vi "Page_Source_WriteShared.vi"(6 "ctlReferences":T1, 7 "top tree items":string[](array[string]), 8 "error in (no error)":errorcluster, 10 "AB_Source in":refnum<class "AB_Source.lvclass">[](array[class]), 11 "AB_PackedLibrary in":refnum<class "AB_PackedLibrary.lvclass">) -> (0 "error out":errorcluster, 2 "AB_Source out":refnum<class "AB_Source.lvclass">[](array[class]), 3 "AB_PackedLibrary out":refnum<class "AB_PackedLibrary.lvclass">)   [LabVIEW 2020, in "AB_PackedLibrary.lvclass"]
uses:
  <vilib>/AppBuilder/AB_Classes/PackedLib/AB_PackedLibrary.lvclass
  e:/builds/penguin/labview/branches/2020/dev/dist/vi.lib/AppBuilder/AB_Classes/Build/AB_Build.lvclass
  e:/builds/penguin/labview/branches/2020/dev/dist/vi.lib/AppBuilder/AB_Classes/TargetFile/AB_Targetfile.lvclass
  <resource>/Framework/Providers/Builds/AppBuilder/AB_UI_Page_Source_Files_References.ctl
  <vilib>/AppBuilder/AB_Classes/Source/AB_Source.lvclass
  <resource>/Framework/Providers/Common/provcom_StringGlobals.vi
  <vilib>/AppBuilder/AB_Classes/Build/AB_Build.lvclass
  <vilib>/AppBuilder/AB_Classes/TargetFile/AB_Targetfile.lvclass
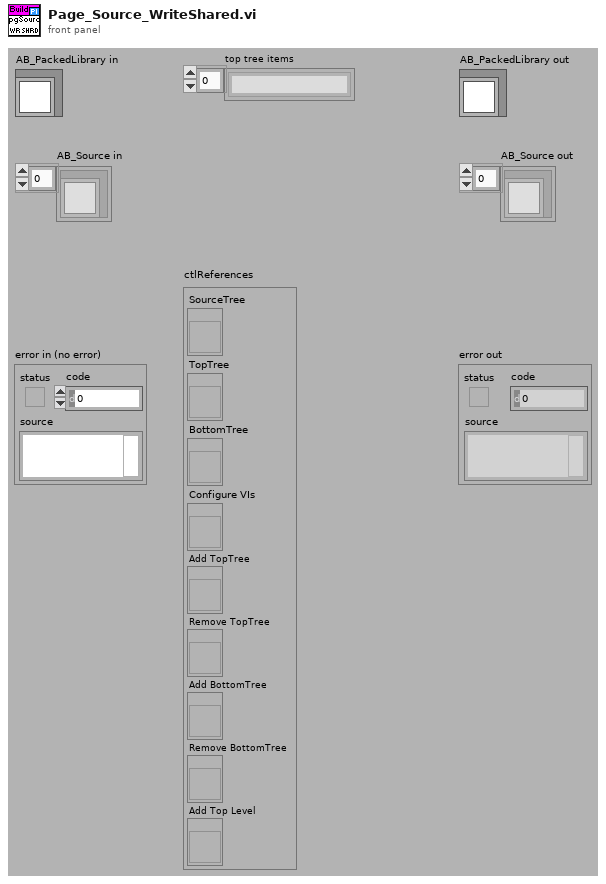
[diagram p1: front panel]
types:
  T1 = typedef "AB_UI_Page_Source_Files_References.ctl" = cluster{"SourceTree":refnum<vi>, "TopTree":refnum<vi>, "BottomTree":refnum<vi>, "Configure VIs":refnum<vi>, "Add TopTree":refnum<vi>, "Remove TopTree":refnum<vi>, "Add BottomTree":refnum<vi>, "Remove BottomTree":refnum<vi>, "Add Top Level":refnum<vi>}
  T2 = typedef "AB_Build.ctl" = cluster{"buildSpecName":string, "buildSpecDescription":string, "destinations":refnum<class "AB_Destination.lvclass">[], "exclusionOption":T3, "defaultLanguage":string, "supportedLanguages":string[], "excludedDirectories":path[], "buildContext":refnum<vi>, "buildObject":T4, "preview":bool, "programatic":bool, "progressBarEvents":T5, "userLog_Path":path, "preActionID":string, "preAction_Path":path, "postActionID":string, "postAction_Path":path, "eng_checkForBrokenVIs?":bool, "eng_verboseLinkerErrors?":bool, "localDest_Path":path, "targetDest_Path":path, "removeVIObject":u16, "cache":refnum<class "PreviewCache.lvclass">, "use cache":bool, "previewCache_ID":string, "buildCache_ID":string, "eng_TempLocalDest_Path":path, "eng_collectDependencies?":bool, "versionInfo":cluster{"buildVersion":cluster{"major":u16, "minor":u16, "patch":u16, "build":u16}, "autoIncrement":bool}, "eng_enableVIChecksums":bool}
  T3 = typedef "AB_Exclusion_Option.ctl" = cluster{"typedefs":bool, "polymorphicVIs":bool, "unusedLibraryItems":bool, "modifyLibraryFile":bool, "edit-timeDependencies":bool, "inlineVIs":bool, "dependent PPLs":bool, "dependent DLLs":bool}
  T4 = typedef "ItemRef.ctl" = u64
  T5 = typedef "provcom_ProgressBar_Events.ctl" = cluster{"newJob":refnum<user-event>, "newItem":refnum<user-event>, "errorMsg":T6, "cancel":refnum<user-event>}
  T6 = typedef "mxLvBuildError.ctl" = refnum<user-event>
  T7 = typedef "AB_Targetfile.ctl" = cluster{"targetfileName":string, "targetfileGUID":string, "enableDebugging":bool, "versionInfo":cluster{"productName":string, "legalCopyright":string, "companyName":string, "internalName":string, "fileDescription":string}, "eng_consolidatedTypeInfo":string, "fastFileFormat":bool, "eng_LEIFBuildData":u32, "versionIndependent":bool}
  T8 = typedef "AB_Source.ctl" = cluster{"path":path, "itemID":string, "parentIndex":i32, "sourceInclusion":T9, "destinationIndex":i32, "properties":T10[], "newName":string, "lvfile":bool, "valid":bool, "eng_inBuild":bool, "eng_isNonVILink":bool, "Amalgamation":bool, "Amalgamation Piece":bool, "eng_delimitedName":string, "preventRename":bool}
  T9 = typedef "AB_Source_Inclusion.ctl" = enum16{"IncludeIfReferenced", "Include", "Exclude", "TopLevel"}
  T10 = typedef "AB_Source_Properties.ctl" = cluster{"sourcePropertyType":T11, "value":variant}
  T11 = typedef "AB_Source_Property_Type.ctl" = enum16{"Remove block diagram", "Remove front panel", "Password", "Window has title bar", "Show menu bar", "Show vertical scroll bar", "Show horizontal scroll bar", "Show toolbar", "Show Abort button", "Show fp when called", "Window behavior", "Allow user to close window", "Window run-time position", "Run when opened", "Allow debugging", "Auto error handling", "Generate guard code", "Use stack variables", "Expression folding", "Integer only", "Inline subVI"}
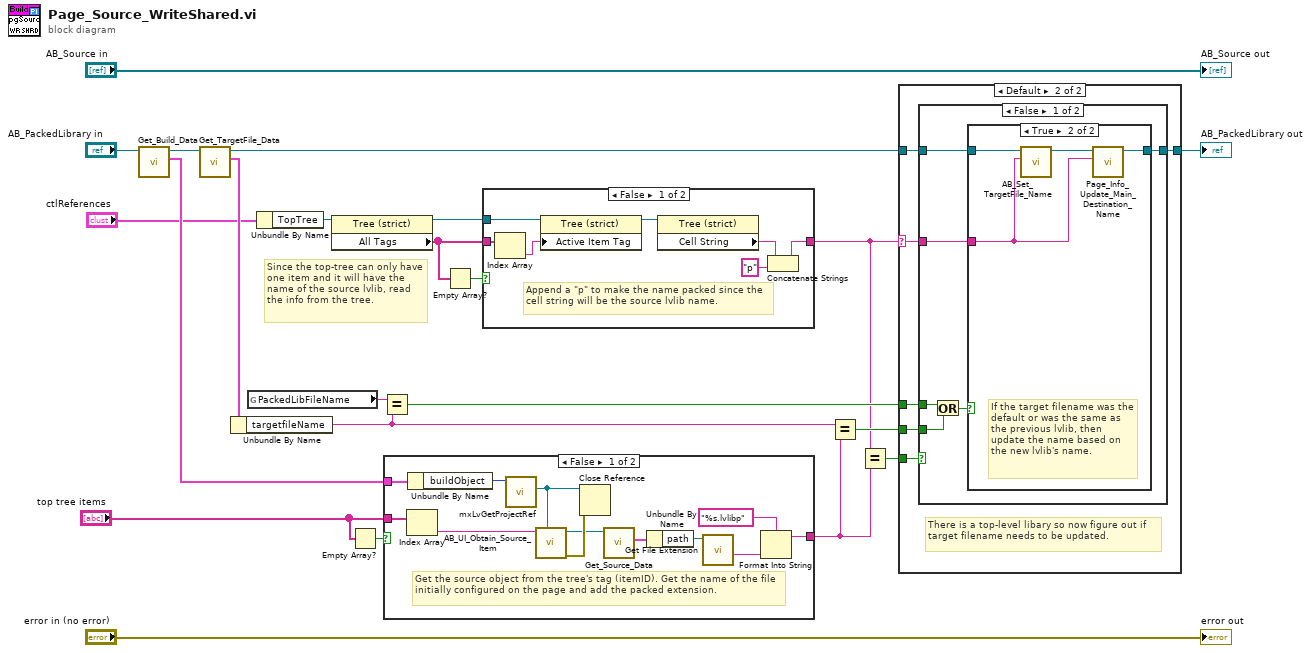
[diagram p0: block diagram]
diagram:
  # "Since the top-tree can only have one item and it will have the name of the source lvlib, read the info from the tree."
  n1 = call <vilib>:"Get_Build_Data.vi"("Class in"="AB_PackedLibrary in") -> ("data"=w18:T2, "Class out"=w17:refnum<class "AB_PackedLibrary.lvclass">)  [unwired: 8 in, 1 out]
  n2 = call <vilib>:"Get_TargetFile_Data.vi"("AB_Targetfile in"=w17) -> ("data"=w16:T7, "AB_Targetfile out"=w7:refnum<class "AB_PackedLibrary.lvclass">)  [unwired: 8 in, 1 out]
  n3 = Unbundle By Name(w16) -> ("targetfileName"=w11:string)
  n4 = global read "provcom_StringGlobals.vi" "PackedLibFileName"() -> (w15:string)
  n5 = Unbundle By Name("ctlReferences") -> ("TopTree"=w4:refnum<vi>)
  n6 = property class="Tree (strict)"(reference=w4) -> (reference out=w3:refnum<vi>, "All Tags"=w2:string[])  [unwired: 1 in, 1 out]
  n7 = Empty Array?(array="top tree items") -> (empty?=w13:bool)
  n8 = Equal?(x=w15, y=w11) -> (x = y?=w12:bool)
  n9 = case shown="False" w13 {
    tunnel: w18 -> [w34 _]
    tunnel: "top tree items" -> [w24 _]
    tunnel: [w23 _] -> w10
    frame False {
      # "Get the source object from the tree's tag (itemID). Get the name of the file initially configured on the page and add the packed extension."
      n10 = Index Array(array=w24) -> (element=w32:string)  [unwired: 1 in]
      n11 = Unbundle By Name(w34) -> ("buildObject"=w33:T4)
      n12 = call <resource>:"mxLvGetProjectRef.vi"("Item"=w33) -> ("Project Refnum"=w30:refnum<vi>)  [unwired: 1 in, 9 out]
      n13 = call <resource>:"AB_UI_Obtain_Source_Item.vi"("Project Refnum"=w30, "source itemID"=w32) -> ("error out"=w31:errorcluster, "source item"=w29:refnum<class "AB_Source.lvclass">)  [unwired: 1 in, 7 out]
      n14 = Close Reference(reference=w30, error in (no error)=w31) -> ()  [unwired: 1 out]
      n15 = call <vilib>:"Get_Source_Data.vi"("Class in"=w29) -> ("data"=w28:T8)  [unwired: 8 in, 2 out]
      n16 = Unbundle By Name(w28) -> ("path"=w25:path)
      n17 = call <vilib>:"Get File Extension.vi"("file"=w25) -> ("filename without extension"=w26:string)  [unwired: 6 in, 4 out]
      n18 = Format Into String(format string="%s.lvlibp", w26) -> (resulting string=w23:string)  [unwired: 2 in, 1 out]
    }
    frame True {
    }
  }
  n19 = Empty Array?(array=w2) -> (empty?=w1:bool)
  n20 = case shown="False" w1 {
    tunnel: w3 -> [w41 _]
    tunnel: [w36 _] -> w6
    tunnel: w2 -> [w35 _]
    frame False {
      # "Append a \"p\" to make the name packed since the cell string will be the source lvlib name."
      n21 = Index Array(array=w35) -> (element=w40:string)  [unwired: 1 in]
      n22 = property class="Tree (strict)"(reference=w41, "Active Item Tag"=w40) -> (reference out=w39:refnum<vi>)  [unwired: 1 in, 1 out]
      n23 = property class="Tree (strict)"(reference=w39) -> ("Cell String"=w37:string)  [unwired: 1 in, 2 out]
      n24 = Concatenate Strings(w37, "p" ("string")) -> (w36:string)
    }
    frame True {
    }
  }
  n25 = Equal?(x=w11, y=w10) -> (x = y?=w9:bool)
  n26 = Equal?(x=w6, y=w10) -> (x = y?=w8:bool)
  n27 = case shown="Default" w6 {
    selector: w6 -> [_ w43]
    tunnel: w12 -> [_ w47]
    tunnel: w9 -> [_ w46]
    tunnel: w8 -> [_ w48]
    tunnel: w7 -> [w42 w45]
    tunnel: [w42 w44] -> w20
    frame "" {
      # "There is no top-level library so do not update anything."
    }
    frame Default {
      # "There is a top-level libary so now figure out if target filename needs to be updated."
      n28 = case shown="False" w48 {
        tunnel: w43 -> [w52 _]
        tunnel: w47 -> [w54 _]
        tunnel: w46 -> [w53 _]
        tunnel: w45 -> [w50 w60]
        tunnel: [w49 w60] -> w44
        frame False {
          n29 = Or(x=w54, y=w53) -> (x .or. y?=w51:bool)
          n30 = case shown="True" w51 {
            tunnel: w52 -> [_ w57]
            tunnel: w50 -> [w55 w58]
            tunnel: [w55 w56] -> w49
            frame False {
              # "The filename was not the default or based on the source lvlib, so don't update."
            }
            frame True {
              # "If the target filename was the default or was the same as the previous lvlib, then update the name based on the new lvlib's name."
              n31 = call <vilib>:"AB_Set_TargetFile_Name.vi"("Target filename"=w57, "TargetFile in"=w58) -> ("TargetFile out"=w59:refnum<class "AB_PackedLibrary.lvclass">)  [unwired: 8 in, 1 out]
              n32 = call-dynamic "Page_Info_Update_Main_Destination_Name.vi"("destination name"=w57, "AB_Build in"=w59) -> ("AB_Build out"=w56:refnum<class "AB_PackedLibrary.lvclass">)  [unwired: 1 in, 8 out]
            }
          }
        }
        frame True {
          # "If the current top-level library is the same as when we entered this page, don't do anything."
        }
      }
    }
  }
  "AB_PackedLibrary out" <- w20
  "error out" <- "error in (no error)"
  "AB_Source out" <- "AB_Source in"
